vi "Test Host Image Acquisition Module.vi"(8 "error in":errorcluster, 11 "Operation":T3) -> (0 "error out":errorcluster, 1 "Image Acquired":bool, 2 "Acq In Progress":bool, 3 "Image":T2(plugin-control))   [LabVIEW 2013]
uses:
  <vilib>/rvi/interface/nirviReadWriteControl/nirviReadWriteControl.xnode
  <vilib>/rvi/interface/nirviMethod/nirviMethod.xnode
  <vilib>/vision/Image Controls.llb/IMAQ Image.ctl
  <vilib>/rvi/interface/nirviCloseFPGA/nirviCloseFPGA.xnode
  Host/FGs/FPGA_Reference.ctl
  Common/CL Configuration.ctl
  Common/CL Signal Mapping.ctl
  Host/Image Acquisition/Image Acquisition Settings FG Enum.ctl
  Host/Image Processing/Mask ROI FG Enum.ctl
  FPGA/Sector/Accumulate/Sector Parameter Cluster.ctl
  Common/Timing/Timing Lib.lvlib
  Host/Globals/Average Sector Data.vi
  Host/System Status/Status FG Enum.ctl
  <vilib>/rvi/errors/niLvFpgaMergeErrorWithErrorCode.vi
  NiFpgaLv.dll
  <vilib>/Utility/error.llb/Error Cluster From Error Code.vi
  <vilib>/rvi/errors/niLvFpgaAdjustHostInterfaceError.vi
  <vilib>/FPGAPlugInAG/PCIe-7842R/niLvFpga_ReadFifo_PCIe-7842R.vi
  FPGA Bitfiles/WingBeatAnalyzer_FPGATargetSim_10_2.lvbitx
  <vilib>/FPGAPlugInAG/PCIe-7842R/niLvFpga_Reset_PCIe-7842R.vi
  <vilib>/FPGAPlugInAG/PCIe-7842R/niLvFpga_Run_PCIe-7842R.vi
  <vilib>/FPGAPlugInAG/PCIe-7842R/niLvFpga_Close_PCIe-7842R.vi
  Host/Image Acquisition/Host Image Acquisition Module Enum.ctl
  Host/Image Acquisition/Acquisition Settings Cluster.ctl
panel:
  out "TO Count":u32
  out "error out 4":errorcluster
  out "error out 5":errorcluster
  out "Actual Depth":u32
  out "Target Sim TO":bool
  out "Cam Data Timeout":bool
  out "Sector FIFO Timeout":bool
  out "Host DMA Timeout":bool
  out "Number of Elements to Write Host DMA":u32
  out "Number of Elements to Read Cam Data":u32
  out "Data":u64[](array[numeric])
  out "Elements Remaining":u32
  out "Words per image":u32
  out "Num Frames read":u32
  out "DMA Words per Image":u32
  out "Acquire":bool
  in  "Acquisition Settings Cluster":T1={"Image Width"=2040, "Image Height"=1088, "Frames To Acquire"=0, "Signal Mapping"=enum."Basler 10-tap", "DMA Buffer Size\n(In Images)"=64} {"Image Height" max=65535; "Image Width" max=65535 step=40}
  out "Buffer Size":u32
  out "Acq'd Frame Width":u32=2040
  out "DMA Write Timeout":bool
  in  "Start Serial Server":bool
  out "Frames Acq'd":u32=1
  out "Acq'd Frame Height":u32=1088
  out "Initialized":bool
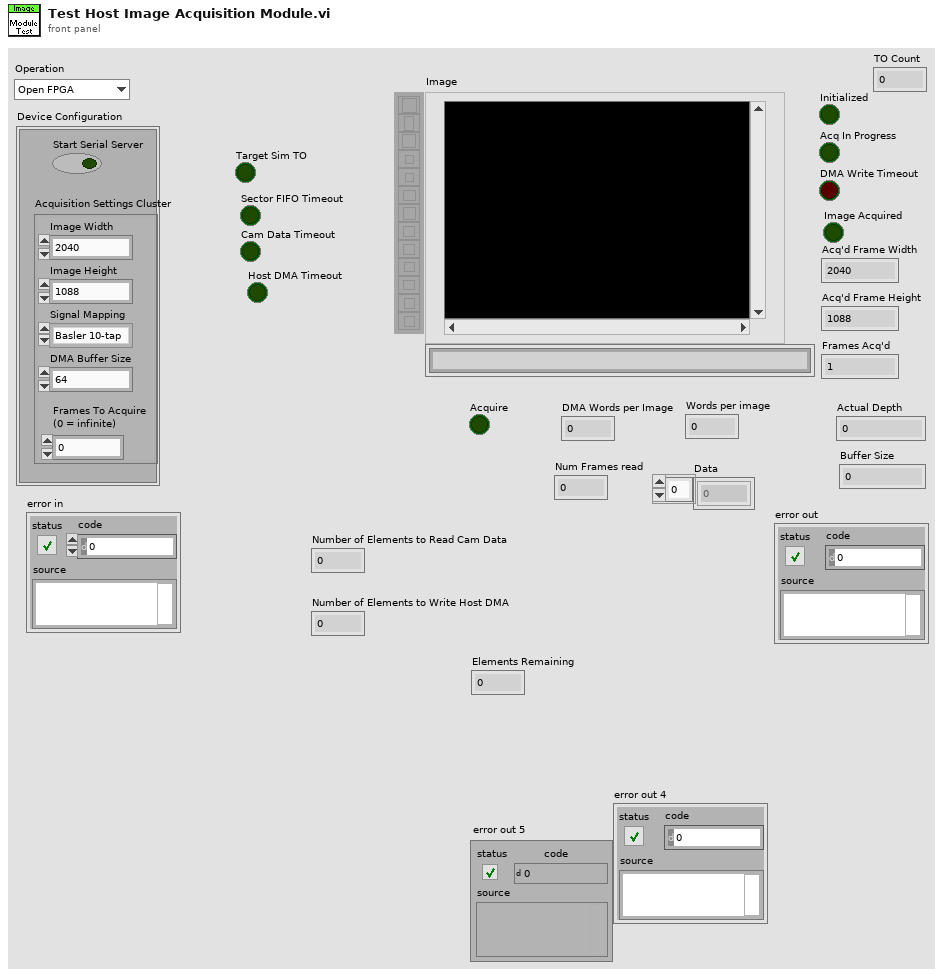
[diagram p1: front panel]
types:
  T1 = typedef "Acquisition Settings Cluster.ctl" = cluster{"Image Width":u32, "Image Height":u32, "Frames To Acquire":u32, "Signal Mapping":enum8{"Standard", "Basler 10-tap", "Vosskühler 10-tap"}, "DMA Buffer Size\n(In Images)":u32}
  T2 = typedef "IMAQ Image.ctl" = refnum<image>
  T3 = typedef "Host Image Acquisition Module Enum.ctl" = enum16{"Open FPGA", "Initialize DMA FIFO", "Load Sim Images", "Initialize Acquisition", "Update Sector Parameters", "Start Acquisition", "Aquire Image", "Read Averages", "Cancel Acquisition", "Close FPGA"}
  T4 = enum8{"Standard", "Basler 10-tap", "Vosskühler 10-tap"}
  T5 = typedef "Image Acquisition Settings FG Enum.ctl" = enum16{"Read", "Write"}
  T6 = typedef "Status FG Enum.ctl" = enum16{"Reset", "Read", "Write"}
  T7 = typedef "Mask ROI FG Enum.ctl" = enum16{"Read", "Write"}
  T8 = typedef "FPGA_Reference.ctl" = refnum<k20>
  T9 = typedef "Image Type" = u32
  T10 = typedef "Mask ROI Cluster.ctl" = cluster{"left annulus":T11, "right annulus":T11, "Threshold Range":cluster{"Lower value":dbl, "Upper value":dbl}, "[Avg BG]":u8[], "Number of Sectors":u8, "Left ROI":T12, "Right ROI":T12, "Left Start Angle Duty Cycle":fxp<+,8,0>, "Left End Angle Duty Cycle":fxp<+,8,0>, "Right End Angle Duty Cycle":fxp<+,8,0>, "Right Start Angle Duty Cycle":fxp<+,8,0>, "[Sector ROIs]":T12[]}
  T11 = typedef "IMAQ Circle" = cluster{"Center X":i32, "Center Y":i32, "Inner Radius":i32, "Outer Radius":i32, "Start Angle":dbl, "End Angle":dbl}
  T12 = typedef "ROI Descriptor" = cluster{"Global Rectangle":i32[], "Contours":cluster{"ID":enum32{"External", "Internal"}, "Type":u32, "Coordinates":i32[]}[]}
  T13 = typedef "Sector Parameter Cluster.ctl" = cluster{"Start Angle":fxp<+/-,17,2>, "End Angle":fxp<+,17,3>, "Inner Radius":u16, "Outter Radius":u16, "Hinge X":u16, "Hinge Y":u16, "NumWingSectors":u8}
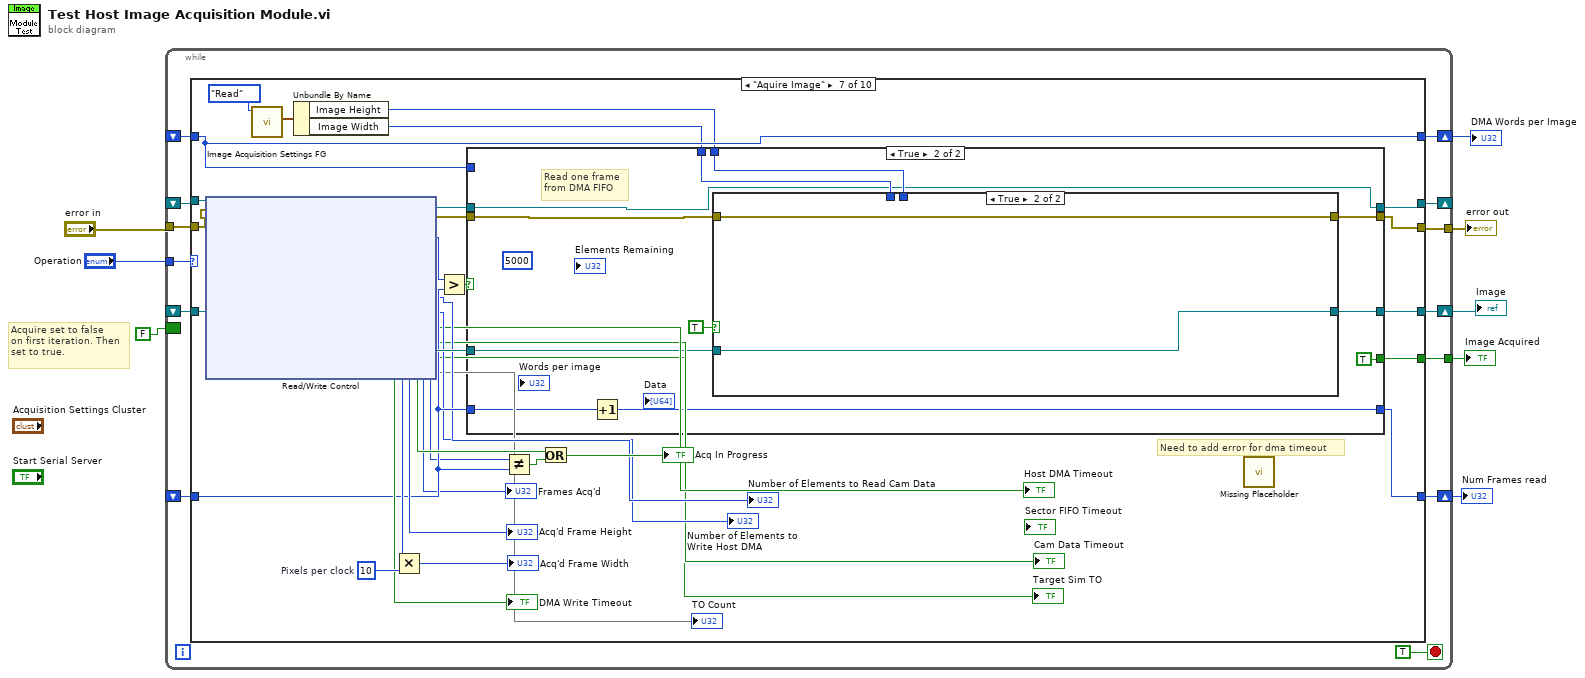
[diagram p0: block diagram]
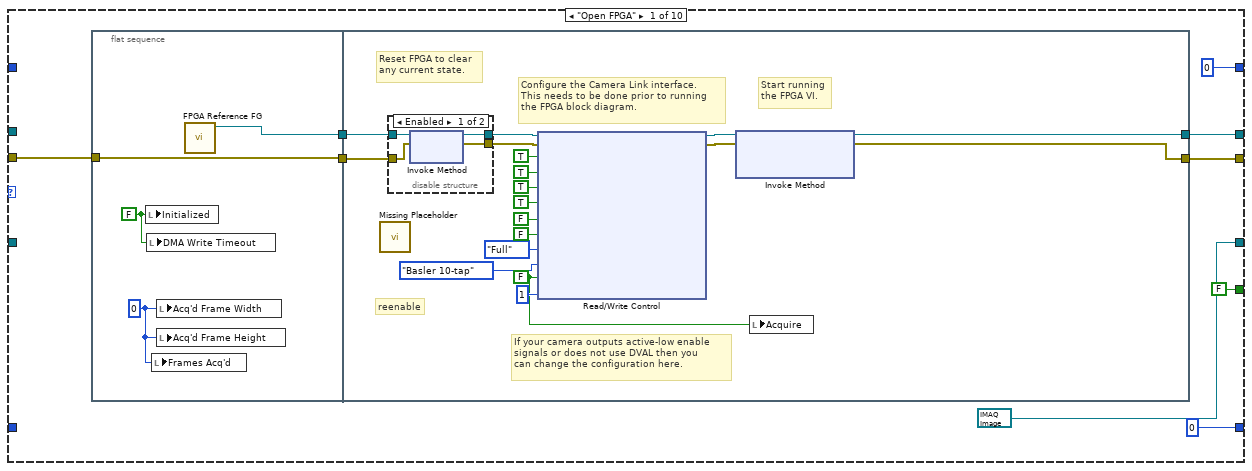
[diagram p2: hidden frame]
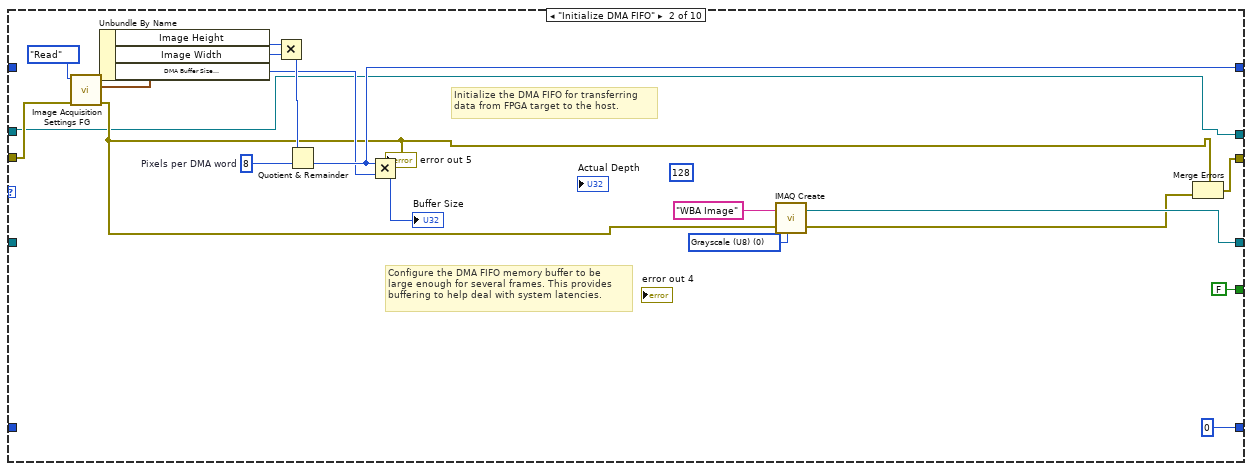
[diagram p4: hidden frame]
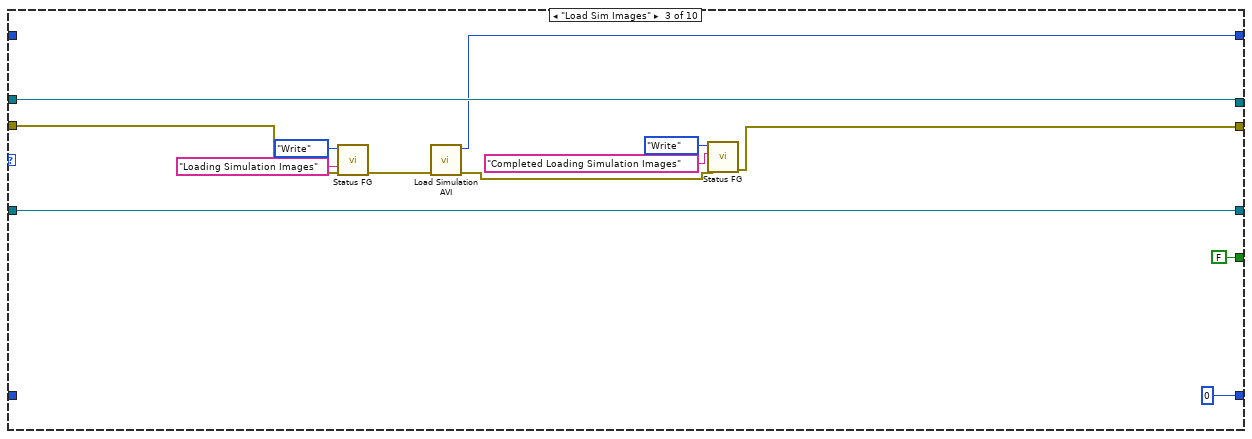
[diagram p5: hidden frame]
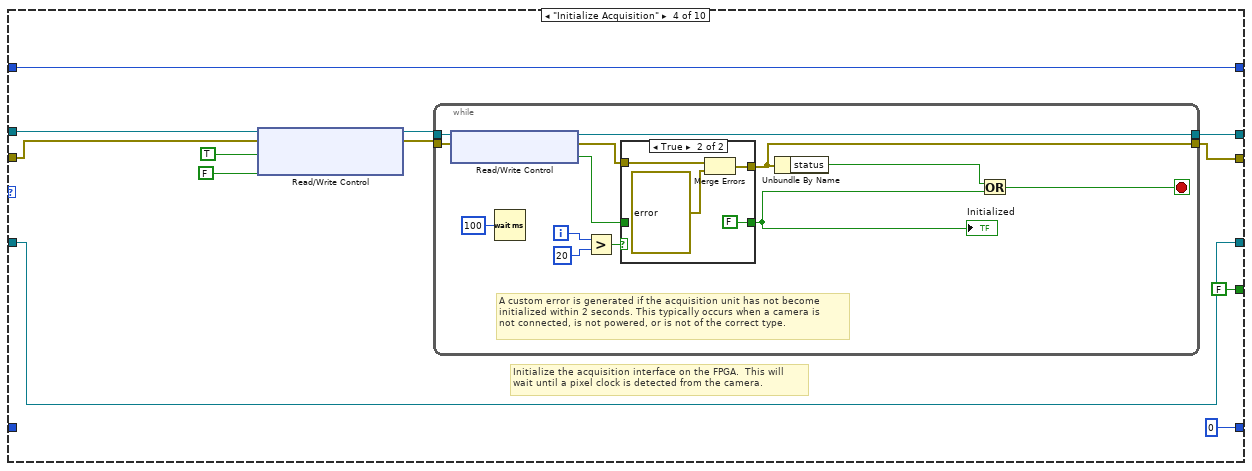
[diagram p6: hidden frame]
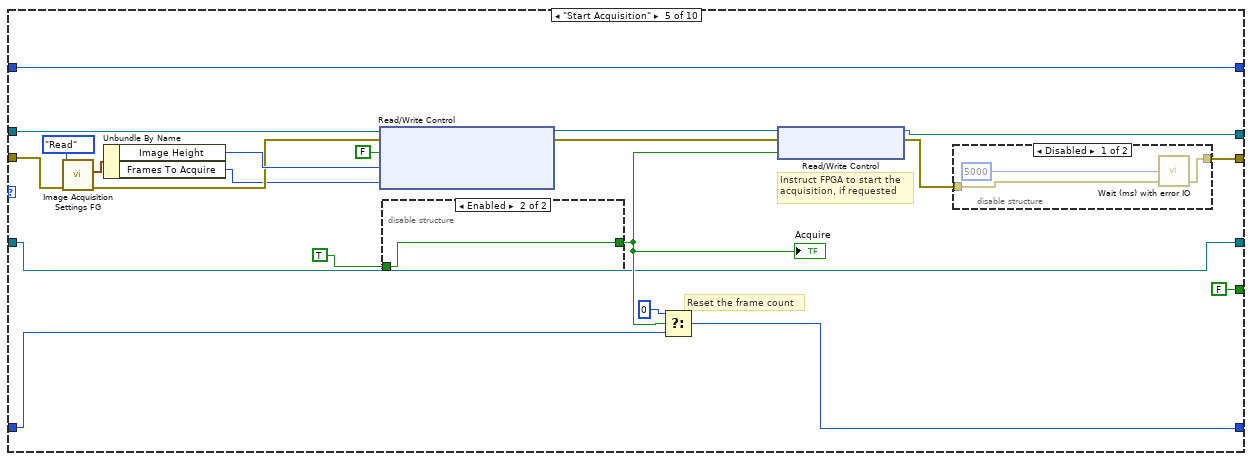
[diagram p8: hidden frame]
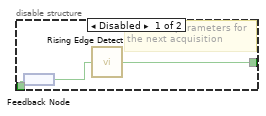
[diagram p10: hidden frame]
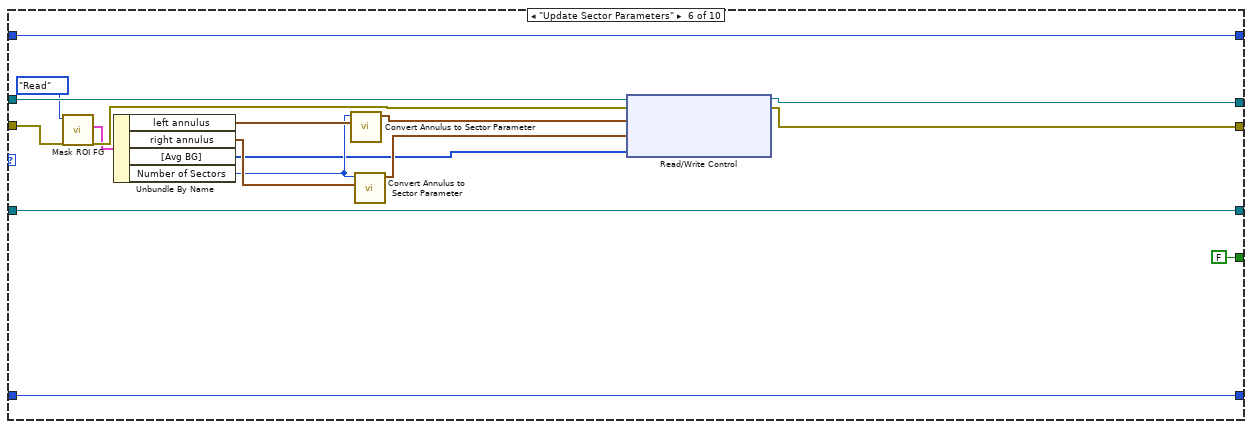
[diagram p11: hidden frame]
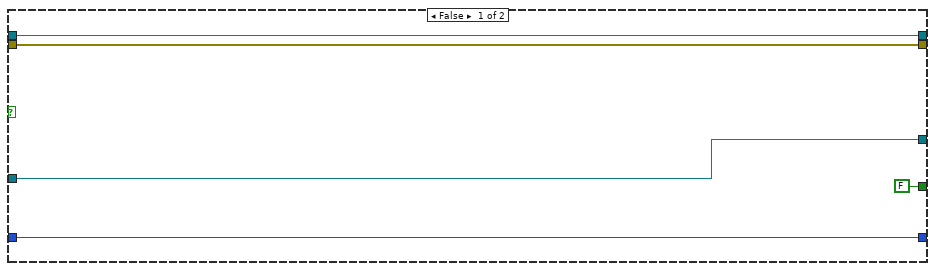
[diagram p12: hidden frame]
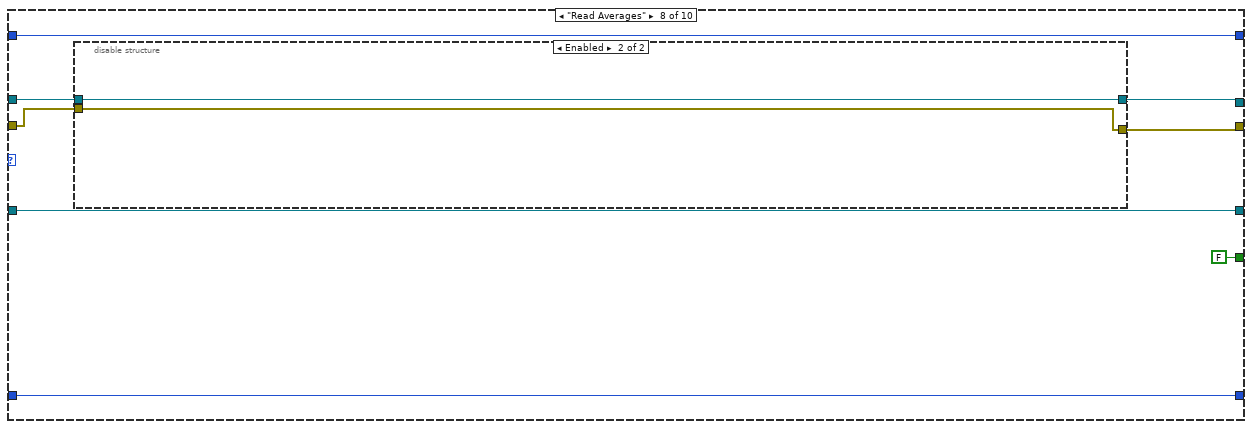
[diagram p14: hidden frame]
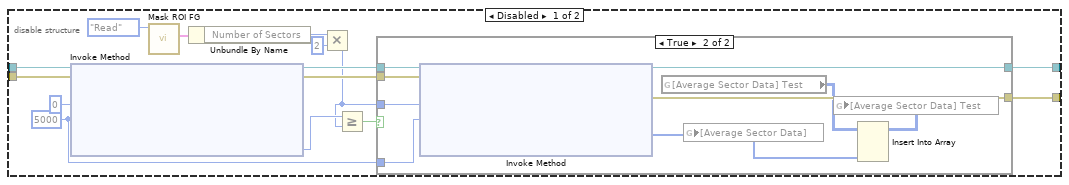
[diagram p15: hidden frame]
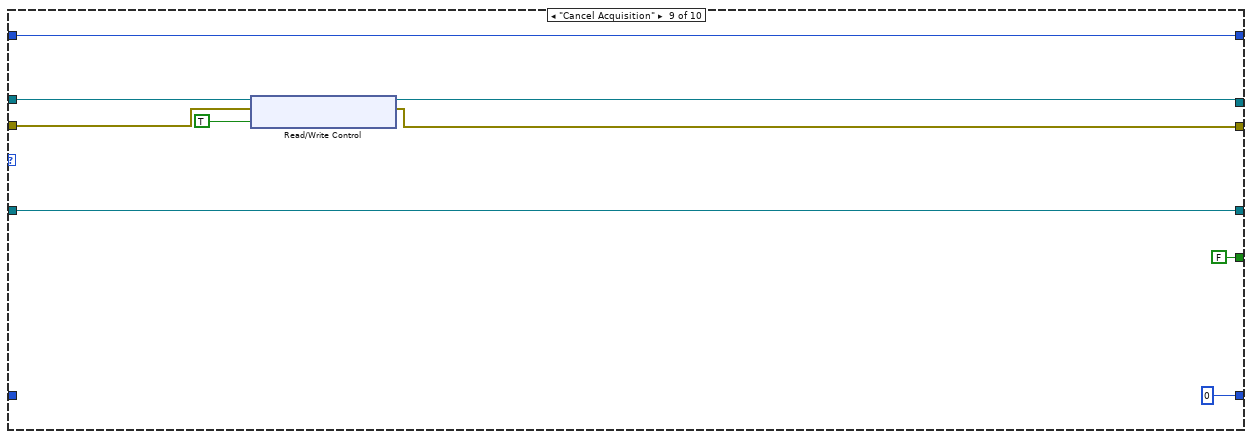
[diagram p17: hidden frame]
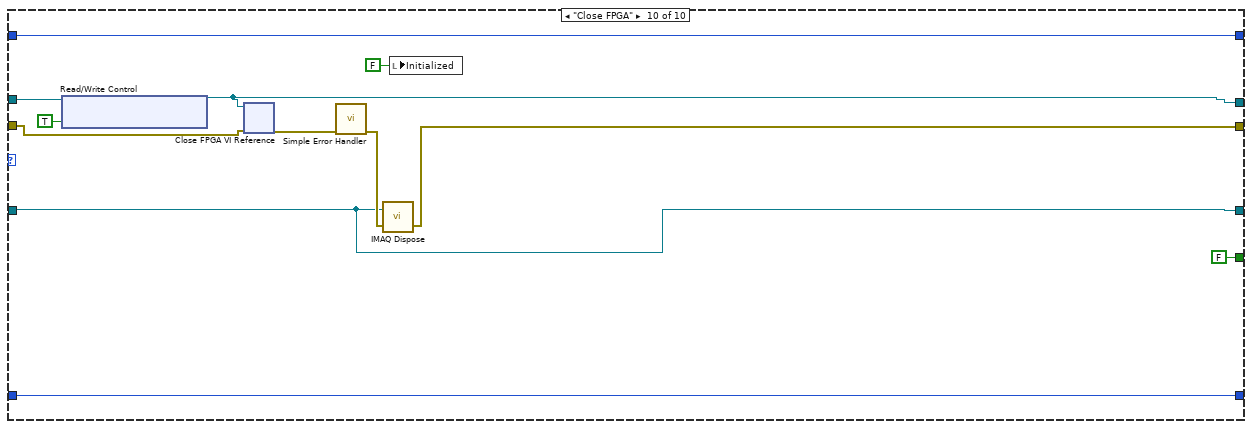
[diagram p18: hidden frame]
diagram:
  # "Acquire set to false\non first iteration. Then\nset to true."
  n1 = while {
    shift-right: [w20] -> _
    shift-left: _ -> [w16]
    tunnel: "error in" -> [w19]
    tunnel: "Operation" -> [w18]
    tunnel: [w17] -> w6
    shift-right: [w15] -> w3
    shift-left: _ -> [w14]
    shift-right: [w13] -> w4
    shift-left: _ -> [w10]
    shift-right: [w12] -> w2
    shift-left: _ -> [w11]
    border: FALSE ("Acquire") -> [_]
    tunnel: [w9] -> w1
    stop <- TRUE stop-if-true
    n2 = case shown="\"Aquire Image\"" w18 {
      tunnel: w19 -> [w30 w67 w85 w92 w135 w165 w180 w220 w260 w266]
      tunnel: [w29 w59 w88 w98 w128 w161 w198 w226 w262 w267] -> w20
      tunnel: [w28 w62 w79 w94 w126 w162 w197 w221 w259 w273] -> w17
      tunnel: w16 -> [_ w59 w88 w99 w136 w167 w199 w227 w264 w269]
      tunnel: [u32 0 w74 w87 w97 w131 w166 w190 w225 w258 w270] -> w15
      tunnel: w14 -> [_ _ _ w97 w131 w166 w190 w225 w258 w270]
      tunnel: [T2 refnum ("New Image") w70 w89 w93 w130 w152 w192 w224 w261 w271] -> w13
      tunnel: [u32 0 u32 0 u32 0 u32 0 w132 w160 w196 w223 u32 0 w272] -> w12
      tunnel: w11 -> [_ _ _ _ w133 w160 w178 w223 _ w272]
      tunnel: w10 -> [_ _ w89 w93 w130 w152 w191 w224 w261 w271]
      tunnel: [FALSE ("Image Acquired") FALSE ("Image Acquired") FALSE ("Image Acquired") FALSE ("Image Acquired") FALSE ("Image Acquired") FALSE ("Image Acquired") w172 FALSE ("Image Acquired") FALSE ("Image Acquired") FALSE ("Image Acquired")] -> w9
      frame "Open FPGA" {
        n3 = flat-sequence {
          tunnel: w30 -> [w31]
          tunnel: [w32] -> w27
          tunnel: [w31] -> w26
          tunnel: [w37] -> w28
          tunnel: [w38] -> w29
          tunnel: w27 -> [w42]
          tunnel: w26 -> [w39]
          frame #0 {
            w33 = u32 0 ("Acq'd Frame Width")
            w34 = FALSE ("Initialized")
            n4 = local write "Initialized"(w34) -> ()
            n5 = local write "DMA Write Timeout"(w34) -> ()
            n6 = local write "Frames Acq'd"(w33) -> ()
            n7 = local write "Acq'd Frame Width"(w33) -> ()
            n8 = local write "Acq'd Frame Height"(w33) -> ()
            n9 = call "FPGA Reference FG.vi"() -> ("FPGA VI Reference Out"=w32:T8)  [unwired: 11 in]
          }
          frame #1 {
            w35 = FALSE ("Acq Control.Acquire")
            # "reenable"
            # "If your camera outputs active-low enable\nsignals or does not use DVAL then you \ncan change the configuration here."
            # "Start running\nthe FPGA VI."
            # "Reset FPGA to clear\nany current state."
            # "Configure the Camera Link interface.\nThis needs to be done prior to running\nthe FPGA block diagram."
            n10 = call "Missing Placeholder.vi"() -> ()  [unwired: 12 in]
            n11 = disable-structure shown="Enabled" {
              disable-tunnel: [w56 w58] -> w46
              disable-tunnel: [w55 w57] -> w44
              disable-tunnel: w42 -> [w54 w58]
              disable-tunnel: w39 -> [w53 w57]
              frame Enabled {
                n12 = xnode "Invoke Method"("FPGA VI Reference In"=w54, "error in"=w53) -> ("FPGA VI Reference Out"=w56:T8, "error out"=w55:errorcluster)
              }
              frame Disabled {
              }
            }
            n13 = xnode "Read/Write Control"("FPGA VI Reference In"=w46, "error in"=w44, "CL Config.FVAL Active High"=TRUE ("IO Module Config.CL FVAL Active High"), "CL Config.LVAL Active High"=TRUE ("IO Module Config.CL LVAL Active High"), "CL Config.DVAL Active High"=TRUE ("IO Module Config.CL DVAL Active High"), "CL Config.Spare Active High"=TRUE ("IO Module Config.CL Spare Active High"), "CL Config.Line Scan"=FALSE, "Acq Control.Ignore DVAL"=FALSE ("CL Config.Line Scan"), "CL Config.Configuration"=enum8{"Base", "Medium", "Full"}."Full", "CL Config.Signal Mapping"=T4."Basler 10-tap", "Acq Control.Acquire"=w35, "# of Frames to Average"=u8 1) -> ("FPGA VI Reference Out"=w43:T8, "error out"=w45:errorcluster)
            n14 = xnode "Invoke Method"("FPGA VI Reference In"=w43, "error in"=w45) -> ("FPGA VI Reference Out"=w38:T8, "error out"=w37:errorcluster)  [unwired: 1 in]
            n15 = local write "Acquire"(w35) -> ()
          }
        }
      }
      frame "Initialize DMA FIFO" {
        (unwired) u32 128 ("Requested Depth")
        w71 = T9 0 items=["Grayscale (U8)", "Grayscale (I16)", "Grayscale (SGL)", "Complex (CSG)", "RGB (U32)", "HSL (U32)", "RGB (U64)", "Grayscale (U16)"] ("Image Type")
        w76 = u32 8  # Pixels per DMA word
        # "Configure the DMA FIFO memory buffer to be\nlarge enough for several frames. This provides\nbuffering to help deal with system latencies."
        # "Initialize the DMA FIFO for transferring\ndata from FPGA target to the host."
        n16 = call "Image Acquisition Settings FG.vi"("error in (no error)"=w67, "Operation"=Image_Acquisition_Settings_FG_Enum."Read") -> ("error out"=w60:errorcluster, "Acquisition Settings Out"=w68:T1)  [unwired: 8 in]
        "error out 5" <- w60
        n17 = Unbundle By Name(w68) -> ("Image Height"=w66:u32, "Image Width"=w65:u32, "DMA Buffer Size\n(In Images)"=w64:u32)
        n18 = Multiply(x=w66, y=w65) -> (x*y=w75:u32)
        n19 = Quotient & Remainder(x=w75, y=w76) -> (floor(x/y)=w74:u32)  [unwired: 1 out]
        n20 = Multiply(x=w74, y=w64) -> (x*y=→"Buffer Size":u32)
        n21 = call "IMAQ Create"("Image Name"="WBA Image", "Image Type"=w71, "error in (no error)"=w60) -> ("New Image"=w70:T2, "error out"=w63:errorcluster)  [unwired: 2 in]
        n22 = Merge Errors(w60, w63) -> (w62:errorcluster)
      }
      frame "Load Sim Images" {
        n23 = call "Status FG.vi"("error in (no error)"=w85, "Status In"="Loading Simulation Images", "Operation"=Status_FG_Enum."Write") -> ("error out"=w84:errorcluster)  [unwired: 7 in, 1 out]
        n24 = call "Load Simulation AVI.vi"("error in (no error)"=w84) -> ("error out"=w80:errorcluster, "Words per image"=w87:u32)  [unwired: 9 in]
        n25 = call "Status FG.vi"("error in (no error)"=w80, "Status In"="Completed Loading Simulation Images", "Operation"=Status_FG_Enum."Write") -> ("error out"=w79:errorcluster)  [unwired: 7 in, 1 out]
      }
      frame "Initialize Acquisition" {
        # "Initialize the acquisition interface on the FPGA.  This will\nwait until a pixel clock is detected from the camera."
        n26 = xnode "Read/Write Control"("FPGA VI Reference In"=w99, "error in"=w92, "Acq Control.Initialize"=TRUE ("Arm Acquisition"), "Acq Control.Cancel Acq"=FALSE) -> ("FPGA VI Reference Out"=w102:T8, "error out"=w101:errorcluster)
        n27 = while {
          tunnel: w102 -> [w111]
          tunnel: w101 -> [w110]
          tunnel: [w109] -> w98
          tunnel: [w112] -> w94
          i -> [w105]
          stop <- w115 stop-if-true
          # "A custom error is generated if the acquisition unit has not become\ninitialized within 2 seconds. This typically occurs when a camera is\nnot connected, is not powered, or is not of the correct type."
          n28 = xnode "Read/Write Control"("FPGA VI Reference In"=w111, "error in"=w110) -> ("FPGA VI Reference Out"=w109:T8, "error out"=w108:errorcluster, "Acq Status.Initialized"=w107:bool)
          n29 = Wait (ms)(milliseconds to wait=u32 100) -> ()  [unwired: 1 out]
          n30 = Greater?(x=w105, y=20) -> (0:w106:bool)
          n31 = case shown="True" w106 {
            tunnel: [w117 FALSE] -> w103
            tunnel: w107 -> [w117 _]
            tunnel: w108 -> [w116 w119]
            tunnel: [w116 w121] -> w112
            frame False {
            }
            frame True {
              n32 = Merge Errors(w119, errorcluster {"status"=TRUE, "code"=-8999, "source"="Acquisition Initialization: This error typically occurs when a camera is not properly connected, is not powered, or is not of the correct type."} ("error in")) -> (w121:errorcluster)
            }
          }
          "Initialized" <- w103
          n33 = Unbundle By Name(w112) -> ("status"=w114:bool)
          n34 = Or(x=w114, y=w103) -> (x .or. y?=w115:bool)
        }
      }
      frame "Start Acquisition" {
        # "Reset the frame count"
        # "Instruct FPGA to start the\nacquisition, if requested"
        n35 = call "Image Acquisition Settings FG.vi"("error in (no error)"=w135, "Operation"=Image_Acquisition_Settings_FG_Enum."Read") -> ("error out"=w134:errorcluster, "Acquisition Settings Out"=w142:T1)  [unwired: 8 in]
        n36 = Unbundle By Name(w142) -> ("Image Height"=w137:u32, "Frames To Acquire"=w124:u32)
        n37 = xnode "Read/Write Control"("FPGA VI Reference In"=w136, "error in"=w134, "Acq Control.Cancel Acq"=FALSE, "Acq Control.Line Scan Height"=w137, "Acq Control.Frames To Acq"=w124) -> ("FPGA VI Reference Out"=w122:T8, "error out"=w123:errorcluster)
        n38 = disable-structure shown="Enabled" {
          disable-tunnel: [w149 w150] -> w139
          disable-tunnel: TRUE ("Acquire") -> [w147 w150]
          frame Disabled {
            # "Write the parameters for\nthe next acquisition"
            n39 = feedback #1() -> (w148:bool)
            n40 = feedback-in #1(w147) -> ()
            n41 = call "Rising Edge Detect.vi"("Input"=w148) -> ("Pulse"=w149:bool)  [unwired: 4 in]
          }
          frame Enabled {
          }
        }
        "Acquire" <- w139
        n42 = Select(t=u32 0, s=w139, f=w133) -> (s? t:f=w132:u32)
        n43 = xnode "Read/Write Control"("FPGA VI Reference In"=w122, "error in"=w123, "Acq Control.Acquire"=w139) -> ("FPGA VI Reference Out"=w128:T8, "error out"=w127:errorcluster)
        n44 = disable-structure shown="Disabled" {
          disable-tunnel: w127 -> [w144 w146]
          disable-tunnel: [w143 w146] -> w126
          frame Disabled {
            n45 = call "Wait (ms) with error IO.vi"("error in (no error)"=w144, "milliseconds to wait"=u32 5000) -> ("error out"=w143:errorcluster)  [unwired: 3 in]
          }
          frame Enabled {
          }
        }
      }
      frame "Update Sector Parameters" {
        n46 = call "Mask ROI FG.vi"("error in (no error)"=w165, "Operation"=Mask_ROI_FG_Enum."Read") -> ("error out"=w164:errorcluster, "Mask ROI Out"=w159:T10)  [unwired: 8 in]
        n47 = Unbundle By Name(w159) -> ("left annulus"=w158:T11, "right annulus"=w156:T11, "[Avg BG]"=w153:u8[], "Number of Sectors"=w155:u8)
        n48 = call "Convert Annulus to Sector Parameter.vi"("Annulus"=w158, "NumWingSectors"=w155) -> ("Sector Parameter"=w157:T13)  [unwired: 9 in]
        n49 = call "Convert Annulus to Sector Parameter.vi"("Annulus"=w156, "NumWingSectors"=w155) -> ("Sector Parameter"=w154:T13)  [unwired: 9 in]
        n50 = xnode "Read/Write Control"("FPGA VI Reference In"=w167, "error in"=w164, "Sector Parameters Left"=w157, "Sector Parameters Right"=w154, "[Average BG Intensity]"=w153) -> ("FPGA VI Reference Out"=w161:T8, "error out"=w162:errorcluster)
      }
      frame "Aquire Image" {
        w188 = u32 10  # Pixels per clock
        # "Need to add error for dma timeout"
        n51 = xnode "Read/Write Control"("FPGA VI Reference In"=w199, "error in"=w180) -> ("FPGA VI Reference Out"=w195:T8, "error out"=w194:errorcluster, "Acq Status.Acq In Progress"=w179:bool, "Acq Status.Frames Acq'd"=w177:u32, "Acq Status.Lines Per Frame"=→"Acq'd Frame Height":u32, "Acq Status.Clocks Per Line"=w187:u32, "Acq Status.DMA Write Timeout"=→"DMA Write Timeout":bool, "Number of Elements to Read Cam Data"=→"Number of Elements to Read Cam Data":u32, "Number of Elements to Write Host DMA"=→"Number of Elements to Write Host DMA":u32, "Host DMA Timeout"=→"Host DMA Timeout":bool, "Cam Data Timeout"=→"Cam Data Timeout":bool, "Target Sim TO"=→"Target Sim TO":bool, "TO Count"=→"TO Count")
        "Frames Acq'd" <- w177
        n52 = call "Image Acquisition Settings FG.vi"("Operation"=Image_Acquisition_Settings_FG_Enum."Read") -> ("Acquisition Settings Out"=w183:T1)  [unwired: 9 in, 1 out]
        n53 = Unbundle By Name(w183) -> ("Image Height"=w182:u32, "Image Width"=w181:u32)
        n54 = Multiply(x=w187, y=w188) -> (x*y=→"Acq'd Frame Width":u32)
        n55 = Greater?(x=w177, y=w178) -> (0:w193:bool)
        n56 = case shown="True" w193 {
          tunnel: w195 -> [w203 w206]
          tunnel: w194 -> [w202 w207]
          tunnel: w182 -> [_ w215]
          tunnel: w181 -> [_ w214]
          tunnel: w191 -> [w204 w213]
          tunnel: [w202 w212] -> w197
          tunnel: [w203 w206] -> w198
          tunnel: w178 -> [w201 w211]
          tunnel: [w201 w210] -> w196
          tunnel: w190 -> [_ _]
          tunnel: [w204 w209] -> w192
          tunnel: [FALSE ("Image Acquired") TRUE ("Image Acquired")] -> w172
          frame False {
          }
          frame True {
            (unwired) 5000 ("Timeout (ms)")
            # "Read one frame\nfrom DMA FIFO"
            n57 = Increment(x=w211) -> (x+1=w210:u32)
            n58 = case shown="True" TRUE {
              tunnel: w215 -> [_ _]
              tunnel: w214 -> [_ _]
              tunnel: w213 -> [w216 w218]
              tunnel: w207 -> [w217 w219]
              tunnel: [w217 w219] -> w212
              tunnel: [w216 w218] -> w209
              frame False {
                # "Do not display the image if we're\nfalling behind in the acquisition."
              }
              frame True {
              }
            }
          }
        }
        n59 = Not Equal?(x=w177, y=w178) -> (x != y?=w176:bool)
        n60 = Or(x=w179, y=w176) -> (x .or. y?=→"Acq In Progress":bool)
        n61 = call "Missing Placeholder.vi"() -> ()  [unwired: 12 in]
      }
      frame "Read Averages" {
        n62 = disable-structure shown="Enabled" {
          disable-tunnel: w227 -> [w242 w255]
          disable-tunnel: [w237 w255] -> w226
          disable-tunnel: [w236 w254] -> w221
          disable-tunnel: w220 -> [w234 w254]
          frame Disabled {
            w238 = 5000 ("Timeout (ms)")
            n63 = xnode "Invoke Method"("FPGA VI Reference In"=w242, "error in"=w234, "Number of Elements"=u32 0, "Timeout (ms)"=w238) -> ("FPGA VI Reference Out"=w240:T8, "error out"=w239:errorcluster, "Elements Remaining"=w230:u32)  [unwired: 1 out]
            n64 = call "Mask ROI FG.vi"("Operation"=Mask_ROI_FG_Enum."Read") -> ("Mask ROI Out"=w233:T10)  [unwired: 9 in, 1 out]
            n65 = Unbundle By Name(w233) -> ("Number of Sectors"=w231:u8)
            n66 = Multiply(x=w231, y=u8 2) -> (x*y=w229:u8)
            n67 = Greater Or Equal?(x=w230, y=w229) -> (x >= y?=w232:bool)
            n68 = case shown="True" w232 {
              tunnel: w240 -> [w244 w253]
              tunnel: w239 -> [w243 w252]
              tunnel: w238 -> [_ w251]
              tunnel: [w244 w250] -> w237
              tunnel: [w243 w249] -> w236
              tunnel: w229 -> [_ w248]
              frame False {
              }
              frame True {
                n69 = xnode "Invoke Method"("FPGA VI Reference In"=w253, "error in"=w252, "Number of Elements"=w248, "Timeout (ms)"=w251) -> ("FPGA VI Reference Out"=w250:T8, "error out"=w249:errorcluster, "Data"=w246:u8[])  [unwired: 1 out]
                n70 = global read "Average Sector Data.vi" "[Average Sector Data] Test"() -> (w247:u8[][])
                n71 = global write "Average Sector Data.vi" "[Average Sector Data]"(w246) -> ()
                n72 = Insert Into Array(array=w247, new element=w246) -> (w245:u8[][])  [unwired: 2 in]
                n73 = global write "Average Sector Data.vi" "[Average Sector Data] Test"(w245) -> ()
              }
            }
          }
          frame Enabled {
          }
        }
      }
      frame "Cancel Acquisition" {
        n74 = xnode "Read/Write Control"("FPGA VI Reference In"=w264, "error in"=w260, "Acq Control.Cancel Acq"=TRUE) -> ("FPGA VI Reference Out"=w262:T8, "error out"=w259:errorcluster)
      }
      frame "Close FPGA" {
        n75 = xnode "Read/Write Control"("FPGA VI Reference In"=w269, "Acq Control.Cancel Acq"=TRUE) -> ("FPGA VI Reference Out"=w267:T8)  [unwired: 1 in, 1 out]
        n76 = xnode "Close FPGA VI Reference"("FPGA VI Reference In"=w267, "error in"=w266) -> ("error out"=w276:errorcluster)
        n77 = call <vilib>:"Simple Error Handler.vi"("error in (no error)"=w276) -> ("error out"=w274:errorcluster)  [unwired: 4 in, 4 out]
        n78 = call "IMAQ Dispose"("Image"=w271, "error in (no error)"=w274) -> ("error out"=w273:errorcluster)  [unwired: 4 in]
        n79 = local write "Initialized"(FALSE ("Initialized")) -> ()
      }
    }
  }
  "error out" <- w6
  "Image" <- w4
  "DMA Words per Image" <- w3
  "Num Frames read" <- w2
  "Image Acquired" <- w1
